vi "Queue Comms Dequeue.vi"(8 "error in":errorcluster) -> (0 "error out":errorcluster, 3 "Data Out":T1={"Estados"=enum."inicio", "Data"=variant}, 5 "queue out":refnum<queue>)   [LabVIEW 2019]
doc: "Este VI saca elementos de la cola."
uses:
  Private Controls/Control HMI Data Cluster.ctl
  Private Controls/Estados.ctl
  Private Controls/Queue FGV Action.ctl
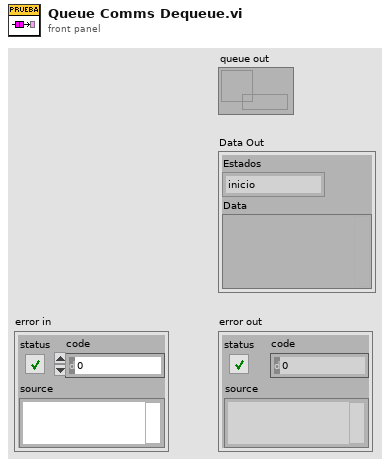
[diagram p1: front panel]
types:
  T1 = typedef "Control HMI Data Cluster.ctl" = cluster{"Estados":T2, "Data":variant}
  T2 = typedef "Estados.ctl" = enum16{"CargaReferencias", "LeerArchivoConfiguracion", "RevisaTipoGenerador", "inicio", "conf_instru", "escribe_frec", "lee_BD", "lee_referencia", "guardarVrefA", "guardarVrefC", "guardarVrefZ", "FrecAmp_A1", "FrecAmp_C1", "FrecAmp_Z1", "FrecAmp_A2", "FrecAmp_C2", "FrecAmp_Z2", "iniciarGEN", "monitoreo", "detenerGEN", "crea_voltajes_prueba_A", "crea_voltajes_prueba_C", "crea_voltajes_prueba_Z", "voltajeInicialA2", "voltajeInicialC2", "voltajeInicialZ2", "actualizarVrefA", "actualizarVrefC", "actualizarVrefZ", "ingresaMedicionesA", "ingresaMedicionesC", "ingresaMedicionesZ", "cumplimiento", "listo_evaluar", "evaluar", "final", "guardaMedicionesA", "guardaMedicionesC", "guardaMedicionesZ", "ultimaFrec", "generaA2", "detieneA2", "salir", "Error"}
  T3 = typedef "Queue FGV Action.ctl" = enum16{"Set", "Get", "Release"}
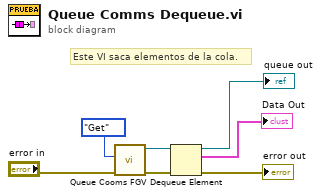
[diagram p0: block diagram]
diagram:
  # "Este VI saca elementos de la cola."
  n1 = call "Queue Cooms FGV.vi"("error in"="error in", "Action"=Queue_FGV_Action."Get") -> ("error out"=w7:errorcluster, "queue out"=w6:refnum<queue>)  [unwired: 8 in]
  n2 = Dequeue Element(queue=w6, error in (no error)=w7) -> (queue out=→"queue out":refnum<queue>, element=→"Data Out":T1, error out=→"error out":errorcluster)  [unwired: 1 in, 1 out]
